vi "NMS.vi"(10 "IoU":sgl=0.45, 11 "Array in":sgl[][](array[numeric])=[[629.96295, 551.19556, 682.1448, 679.6157, 0.978765], [630.6488, 551.74133, 682.2727, 680.2747, 0.985854], [630.00916, 551.4957, 681.65173, 679.59985, 0.983157], [630.68286, 551.3997, 681.5454, 679.5936, 0.987858], [631.0, 552.2371, 682.35455, 679.66736, 0.983014], [630.0213, 552.1413, 681.43494, 679.5249, 0.986384], [631.01324, 551.53723, 680.9933, 679.8141, 0.986177], [631.23315, 551.2095, 682.34, 680.6802, 0.982225], [630.0841, 551.2878, 681.771, 680.8048, 0.983458], [631.1553, 551.02734, 680.6134, 681.4035, 0.986422]]) -> (3 "Box out":T1[](array[typedef]))   [LabVIEW 2017, in "process_YOLOv8.lvlib"]
uses:
  process_YOLOv8.lvlib
  Box.ctl
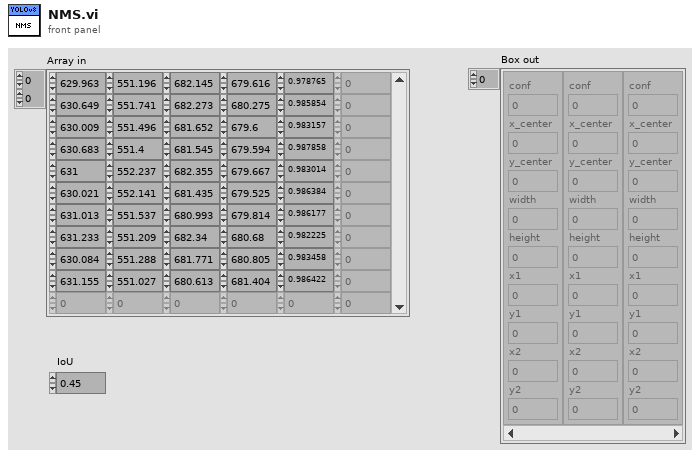
[diagram p1: front panel]
types:
  T1 = typedef "process_YOLOv8.lvlib/Box.ctl" = cluster{"conf":sgl, "x_center":sgl, "y_center":sgl, "width":sgl, "height":sgl, "x1":sgl, "y1":sgl, "x2":sgl, "y2":sgl}
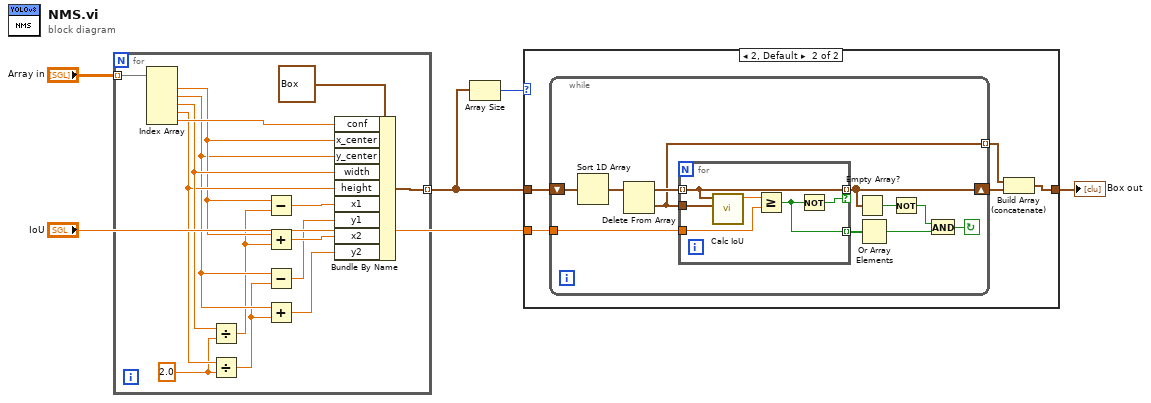
[diagram p0: block diagram]
diagram:
  n1 = for {
    tunnel: "Array in" -> [w20] mode=indexing
    tunnel: [w7] -> w2 mode=indexing
    w16 = sgl 2.0 ("y")
    n2 = Index Array(array=w20) -> (element #1=w14:sgl, element #2=w12:sgl, element #3=w18:sgl, element #4=w17:sgl, element #5=w19:sgl)  [unwired: 5 in]
    n3 = Divide(x=w18, y=w16) -> (x/y=w11:sgl)
    n4 = Divide(x=w17, y=w16) -> (x/y=w10:sgl)
    n5 = Subtract(x=w14, y=w11) -> (x-y=w15:sgl)
    n6 = Add(x=w14, y=w11) -> (x+y=w13:sgl)
    n7 = Subtract(x=w12, y=w10) -> (x-y=w9:sgl)
    n8 = Add(x=w12, y=w10) -> (x+y=w8:sgl)
    n9 = Bundle By Name(cluster=T1 {"conf"=0.0, "x_center"=0.0, "y_center"=0.0, "width"=0.0, "height"=0.0, "x1"=0.0, "y1"=0.0, "x2"=0.0, "y2"=0.0}, "conf"=w19, "x_center"=w14, "y_center"=w12, "width"=w18, "height"=w17, "x1"=w15, "y1"=w9, "x2"=w13, "y2"=w8) -> (w7:T1)
  }
  n10 = Array Size(array=w2) -> (size(s)=w1:i32)
  n11 = case shown="2, Default" w1 {
    tunnel: "IoU" -> [_ w26]
    tunnel: [w21 w23] -> w3
    tunnel: w2 -> [w21 w24]
    frame 0, 1 {
    }
    frame 2, Default {
      n12 = while {
        shift-right: [w29] -> w25
        shift-left: w24 -> [w37]
        tunnel: w26 -> [w34]
        tunnel: [w32] -> w22 mode=indexing
        stop <- w30 continue-if-true
        n13 = Sort 1D Array(array=w37) -> (sorted array=w36:T1[])
        n14 = Delete From Array(array=w36) -> (deleted portion=w32:T1, array with subset deleted=w35:T1[])  [unwired: 2 in]
        n15 = for {
          tunnel: w35 -> [w40] mode=indexing
          tunnel: w32 -> [w43]
          tunnel: w34 -> [w41]
          tunnel: [w40] -> w29 mode=indexing if=w39
          tunnel: [w38] -> w33 mode=indexing
          n16 = call "Calc IoU.vi"("Box_2"=w43, "Box_1"=w40) -> ("IoU"=w42:sgl)  [unwired: 9 in]
          n17 = Greater Or Equal?(x=w42, y=w41) -> (x >= y?=w38:bool)
          n18 = Not(x=w38) -> (.not. x?=w39:bool)
        }
        n19 = Empty Array?(array=w29) -> (empty?=w28:bool)
        n20 = Or Array Elements(Boolean array=w33) -> (logical OR=w31:bool)
        n21 = Not(x=w28) -> (.not. x?=w27:bool)
        n22 = And(x=w27, y=w31) -> (x .and. y?=w30:bool)
      }
      n23 = Build Array (concatenate)(w22, w25) -> (w23:T1[])
    }
  }
  "Box out" <- w3
